vi "Draw Text.vi"(4 "Text Format":refnum<k24>, 5 "Encoding":refnum<k24>, 6 "Brush":refnum<k24>, 7 "Font":refnum<k24>, 8 "error in (no error)":errorcluster, 9 "Offset":cluster{"x":sgl, "y":sgl}, 10 "Bytes":u8[](array[numeric]), 11 "Canvas in":refnum<class "Drawer .Net.lvclass">) -> (0 "error out":errorcluster, 3 "Canvas out":refnum<class "Drawer .Net.lvclass">)   [LabVIEW 2023, in "Glyph .NET Drawer.lvlib" / "Drawer .Net.lvclass"]
uses:
  Drawer .Net.lvclass
  System.Drawing
  Drawer .Net.lvclass/Drawer .Net.ctl
  E:/Labview/LV 2023/Libs/LV Symbol/Glyph .NET Drawer/LVFont.dll
  LVFont.dll
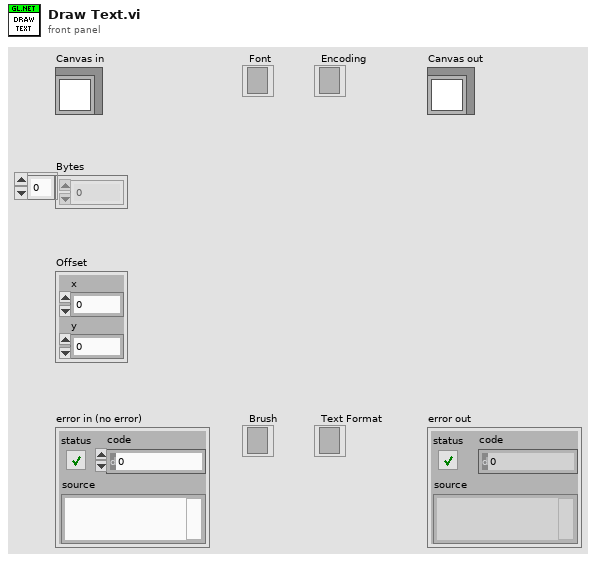
[diagram p1: front panel]
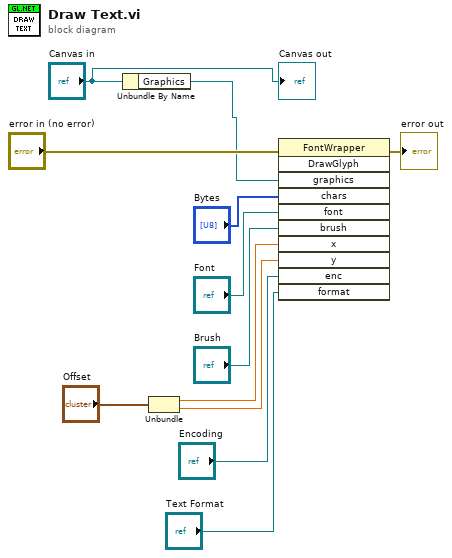
[diagram p0: block diagram]
diagram:
  n1 = Unbundle By Name("Canvas in") -> ("Graphics"=w2:refnum<k24>)
  n2 = Unbundle("Offset") -> ("x"=w11:sgl, "y"=w12:sgl)
  n3 = invoke class="FontWrapper" method="DrawGlyph"(error in="error in (no error)", "graphics"=w2, "chars"="Bytes", "font"="Font", "brush"="Brush", "x"=w11, "y"=w12, "enc"="Encoding", "format"="Text Format") -> (error out=→"error out":errorcluster)  [unwired: 2 in, 10 out]
  "Canvas out" <- "Canvas in"
